vi "Estación-meteorologica.vi"() -> ()   [LabVIEW 2016]
uses:
  <vilib>/MakerHub/LINX/Public/Peripherals/Analog/Analog Read N Chans.vi
  <vilib>/MakerHub/LINX/Private/Local IO/LinxAnalogRead.vi
  <vilib>/MakerHub/LINX/Public/Utilities/Check Channel.vi
  <vilib>/MakerHub/LINX/Public/Utilities/Open Serial.vi
  <vilib>/MakerHub/LINX/Private/Utilties/Generate Error.vi
  <vilib>/MakerHub/LINX/LMH-LINX.lvlib
panel:
  out "Luminosidad":dbl(graph)
  out "Temperatura":dbl(graph)
  out "Luminosidad":u8(knob) scale=0.0..100.0
  out "Alerta alta Tª":bool
  out "Alerta baja Tª":bool
  out "Alerta Lluvia":bool
  out "LLuvia":dbl(slide) scale=0.0..100.0
  out "Temperatura":dbl(slide) scale=0.0..50.0
  in  "AI Channel(s)":u8[](array[numeric])
  in  "Baud Rate Override":u32
  in  "stop":bool
  in  "Serial Port":refnum<visa-resource-name>="N/A"
  # "Estación Metereológica"
  # "Configuración"
  # "Víctor Galvín Coronil"
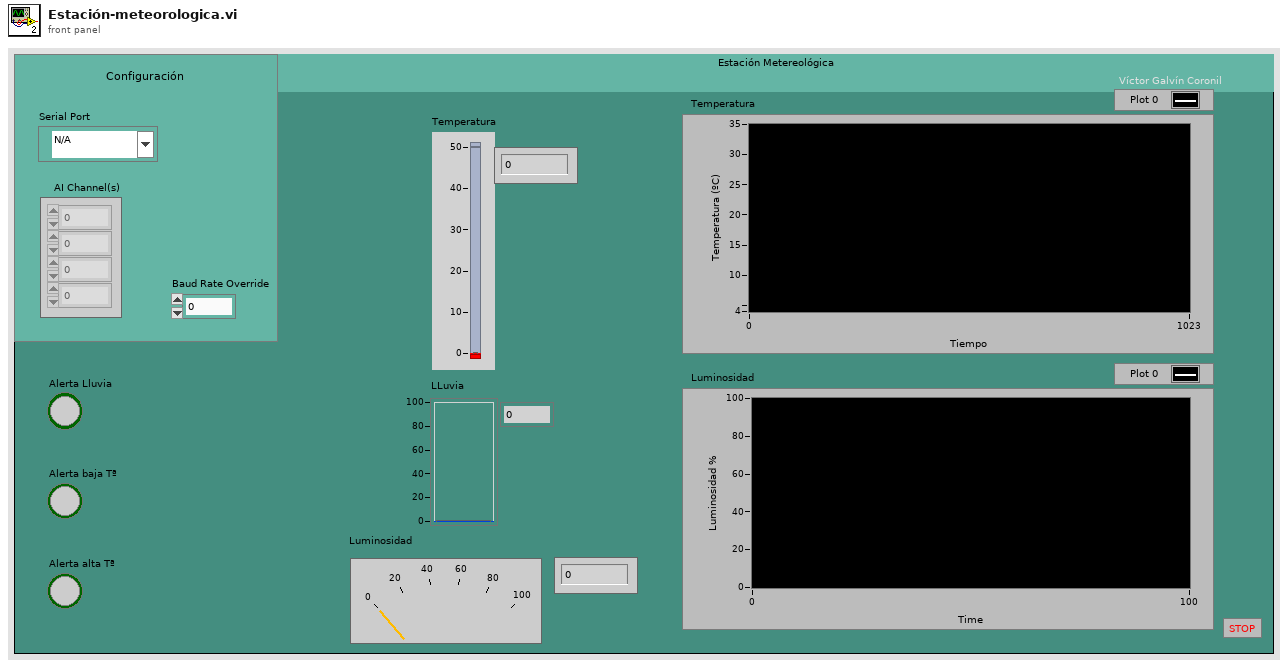
[diagram p1: front panel]
types:
  T1 = typedef "LMH-LINX.lvlib/LINX Ref.ctl" = cluster{"IO":T2, "Interface":T3, "LINX Device Config":T4}
  T2 = typedef "LMH-LINX.lvlib/Platform.ctl" = enum16{"Remote", "Local"}
  T3 = typedef "LMH-LINX.lvlib/Interface.ctl" = enum16{"Serial", "TCP"}
  T4 = typedef "LMH-LINX.lvlib/Device.lvlib/LINX Device Config.ctl" = cluster{"Interface":T3, "COM Port":refnum<visa-resource-name>, "TCP Configuration":T5, "Device Family":u8, "Device ID":u8, "Device Name":string, "TCP Ref":refnum<k5>, "Channels":T6}
  T5 = typedef "LMH-LINX.lvlib/Device.lvlib/TCP Config.ctl" = cluster{"IP Address":string, "Port":u16}
  T6 = typedef "LMH-LINX.lvlib/Channels.ctl" = cluster{"DI":u8[], "DO":u8[], "AI":u8[], "AO":u8[], "PWM":u8[], "QE":u8[], "UART":u8[], "I2C 2":u8[], "SPI":u8[], "CAN":u8[], "Servo":u8[], "AI Ref (V)":dbl, "AI Resolution (Bits)":u8, "AO Ref (V)":dbl, "AO Resolution (Bits)":u8}
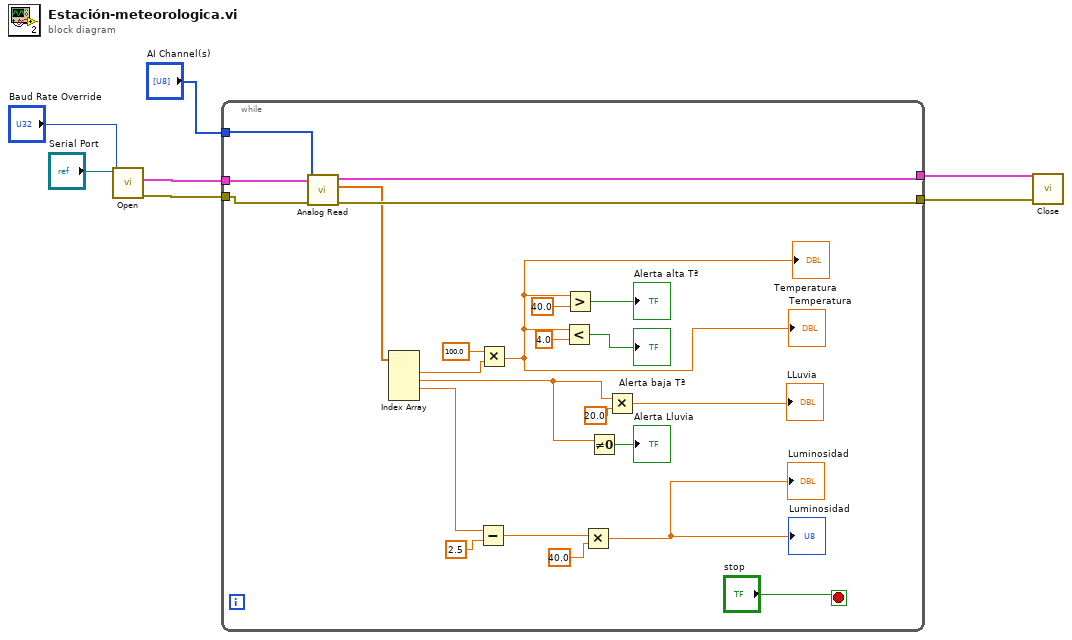
[diagram p0: block diagram]
diagram:
  n1 = call-poly <vilib>:"Open.vi"("Baud Rate Override"="Baud Rate Override", "Serial Port"="Serial Port") -> ("Error Out"=w4:errorcluster, "LINX Resource"=w6:T1)  [unwired: 7 in, 1 out]
  n2 = while {
    tunnel: w6 -> [w20]
    tunnel: [w30] -> w5
    tunnel: w4 -> [w19]
    tunnel: [w29] -> w1
    tunnel: "AI Channel(s)" -> [w27]
    stop <- "stop" stop-if-true
    n3 = call-poly <vilib>:"Analog Read.vi"("Error In"=w19, "AI Channel(s)"=w27, "LINX Resource"=w20) -> ("Error Out"=w29:errorcluster, "Voltages"=w18:dbl[], "LINX Resource"=w30:T1)  [unwired: 5 in, 1 out]
    n4 = Index Array(array=w18) -> (element #1=w17:dbl, element #2=w10:dbl, element #3=w12:dbl)  [unwired: 4 in, 1 out]
    n5 = Subtract(x=w12, y=2.5) -> (x-y=w11:dbl)
    n6 = Multiply(x=100.0, y=w17) -> (x*y=w16:dbl)
    "Temperatura" <- w16
    "Temperatura" <- w16
    n7 = Less?(x=w16, y=4.0) -> (x < y?=→"Alerta baja Tª":bool)
    n8 = Greater?(x=w16, y=40.0) -> (0:→"Alerta alta Tª":bool)
    n9 = Multiply(x=w11, y=40.0) -> (x*y=→"Luminosidad" →"Luminosidad":dbl)
    n10 = Not Equal To 0?(x=w10) -> (x != 0?=→"Alerta Lluvia":bool)
    n11 = Multiply(x=w10, y=20.0) -> (x*y=→"LLuvia":dbl)
  }
  n12 = call <vilib>:"Close.vi"("Error In"=w1, "LINX Resource"=w5) -> ()  [unwired: 9 in, 1 out]
